vi "Test TDMS.vi"() -> ()   [LabVIEW 2020]
uses:
  Labview Library/Libraries/Basic Experiment/T1 Settings.ctl
  Labview Library/Libraries/Basic Experiment/Basic Experiment.lvlib
panel:
  in  "file path":path
  in  "T1 Settings":T1={"Pi(s)"=1.2e-07, "Loop Per Update"=1000, "Update Times"=10, "MW Fre"=1350.0, "MW Power"=-27.0, "Tau Start"=1e-08, "Tau End"=0.0002, "Num"=40, "AutoTrace Before Exp"=TRUE} {"Tau End" format="%#_6p"; "Tau Start" format="%#_6p"; "Pi(s)" format="%#_6p"}
  # "T1 Settings"
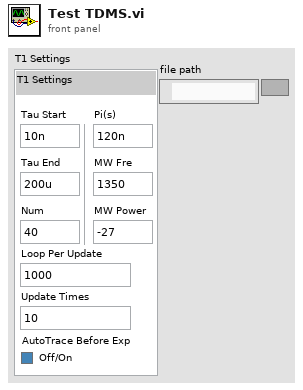
[diagram p1: front panel]
types:
  T1 = typedef "Basic Experiment.lvlib/T1 Settings.ctl" = cluster{"Pi(s)":dbl, "Loop Per Update":u32, "Update Times":u32, "MW Fre":dbl, "MW Power":dbl, "Tau Start":dbl, "Tau End":dbl, "Num":u32, "AutoTrace Before Exp":bool}
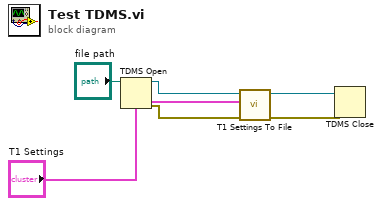
[diagram p0: block diagram]
diagram:
  n1 = TDMS Open(11:"file path") -> (0:w5:errorcluster, 3:w6:refnum<k34>)  [unwired: 6 in]
  n2 = call "T1 Settings To File.vi"("error in (no error)"=w5, "T1 Settings"="T1 Settings", "tdms file"=w6) -> ("error out"=w3:errorcluster, "tdms file out"=w4:refnum<k34>)  [unwired: 7 in]
  n3 = TDMS Close(8:w3, 11:w4) -> ()  [unwired: 2 out]
